vi "Move Stage.vi"() -> ()   [LabVIEW 2016]
uses:
  C:/Program Files/Newport/Piezo Motion Control/Newport AG-UC2-UC8 Applet/Samples/LabVIEW 2009/AgilisCmdLib.dll
  Program Files/Newport/Piezo Motion Control/Newport AG-UC2-UC8 Applet/Samples/LabVIEW 2009/AgilisCmdLib.dll
panel:
  in  "Step speed":i64(ring)=3 items=["Off", "Slow", "Medium", "Fast"]
  in  "Direction":bool
  in  "stop GUI":bool
  in  "Go!":bool
  in  "Stage Address":i32(ring)=3 items=["Dropper"=3, "opposite to dropper"=1, "beside dropper"=2]
  out "error out":errorcluster
  # "In"
  # "Out"
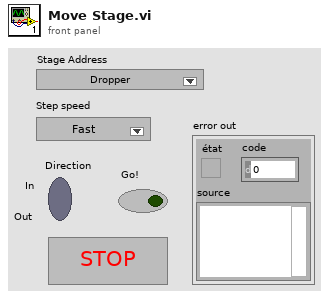
[diagram p1: front panel]
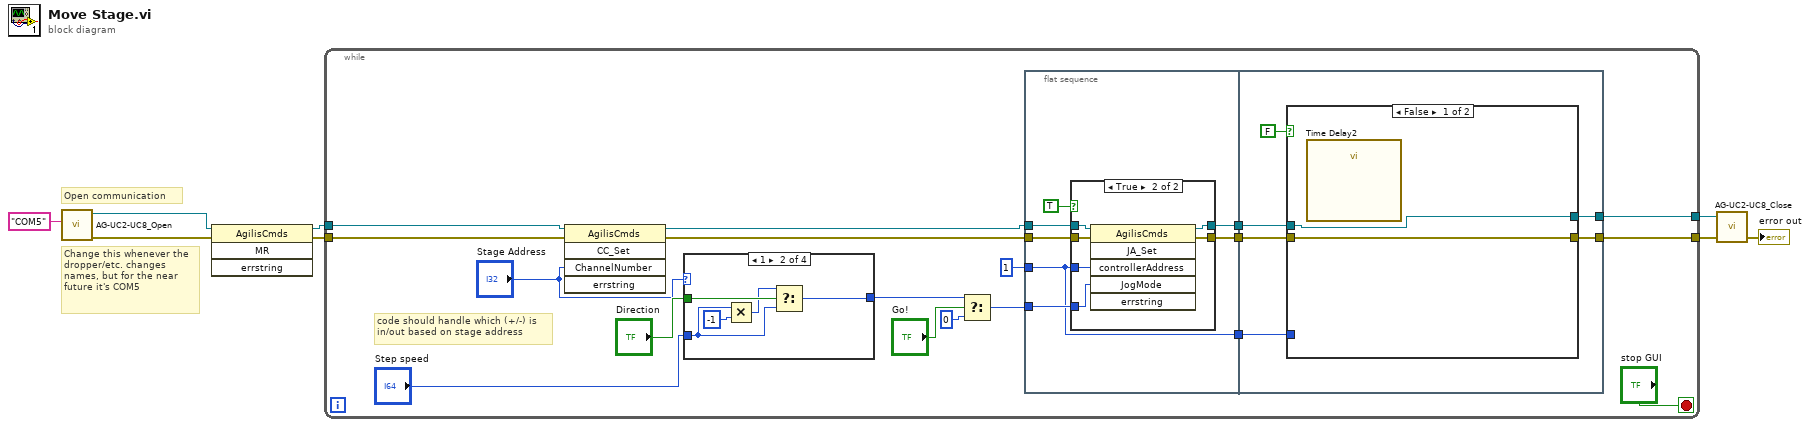
[diagram p0: block diagram]
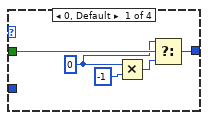
[diagram p2: hidden frame]
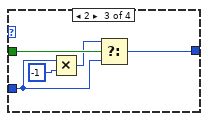
[diagram p3: hidden frame]
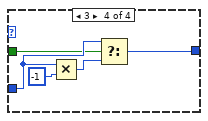
[diagram p4: hidden frame]
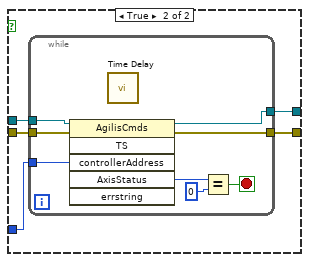
[diagram p6: hidden frame]
diagram:
  # "Change this whenever the dropper/etc. changes names, but for the near future it's COM5"
  # "Open communication"
  n1 = call "AG-UC2-UC8_Open.vi"("Instrument Key IN"="COM5") -> ("error out"=w2:errorcluster, "AG-UC2-UC8 Reference"=w3:refnum<k24>)  [unwired: 3 in, 2 out]
  n2 = invoke class="AgilisCmds" method="MR"(reference=w3, error in=w2) -> (reference out=w4:refnum<k24>, error out=w5:errorcluster)  [unwired: 2 in, 2 out]
  n3 = while {
    tunnel: [w23] -> w7
    tunnel: [w22] -> w6
    tunnel: w4 -> [w17]
    tunnel: w5 -> [w16]
    stop <- "stop GUI" stop-if-true
    # "code should handle which (+/-) is in/out based on stage address"
    n4 = invoke class="AgilisCmds" method="CC_Set"(reference=w17, error in=w16, "ChannelNumber"="Stage Address") -> (reference out=w15:refnum<k24>, error out=w14:errorcluster)  [unwired: 2 in, 3 out]
    n5 = case shown="1" "Stage Address" {
      tunnel: "Step speed" -> [_ w33 w37 w46]
      tunnel: [w29 w35 w39 w43] -> w9
      tunnel: "Direction" -> [w30 w34 w40 w44]
      frame 0, Default {
        w27 = i64 0 ("y")
        n6 = Multiply(x=w27, y=i64 -1) -> (x*y=w28:i32)
        n7 = Select(t=w27, s=w30, f=w28) -> (s? t:f=w29:i64)
      }
      frame 1 {
        n8 = Multiply(x=w33, y=i64 -1) -> (x*y=w32:i32)
        n9 = Select(t=w32, s=w34, f=w33) -> (s? t:f=w35:i64)
      }
      frame 2 {
        n10 = Multiply(x=w37, y=i64 -1) -> (x*y=w38:i32)
        n11 = Select(t=w38, s=w40, f=w37) -> (s? t:f=w39:i64)
      }
      frame 3 {
        n12 = Multiply(x=w46, y=i64 -1) -> (x*y=w42:i32)
        n13 = Select(t=w46, s=w44, f=w42) -> (s? t:f=w43:i64)
      }
    }
    n14 = Select(t=w9, s="Go!", f=i64 0) -> (s? t:f=w18:i64)
    n15 = flat-sequence {
      tunnel: w14 -> [w53]
      tunnel: w15 -> [w52]
      tunnel: 1 ("controllerAddress") -> [w48]
      tunnel: w18 -> [w51]
      tunnel: [w50] -> w26
      tunnel: [w49] -> w25
      tunnel: [w48] -> w21
      tunnel: w26 -> [w67]
      tunnel: w25 -> [w66]
      tunnel: [w65] -> w23
      tunnel: [w64] -> w22
      tunnel: w21 -> [w63]
      frame #0 {
        n16 = case shown="True" TRUE {
          tunnel: w53 -> [w54 w61]
          tunnel: w52 -> [w55 w60]
          tunnel: w48 -> [_ w59]
          tunnel: w51 -> [_ w56]
          tunnel: [w55 w58] -> w50
          tunnel: [w54 w57] -> w49
          frame False {
          }
          frame True {
            n17 = invoke class="AgilisCmds" method="JA_Set"(reference=w60, error in=w61, "controllerAddress"=w59, "JogMode"=w56) -> (reference out=w58:refnum<k24>, error out=w57:errorcluster)  [unwired: 2 in, 4 out]
          }
        }
      }
      frame #1 {
        n18 = case shown="False" FALSE {
          tunnel: w67 -> [w69 w74]
          tunnel: w66 -> [w68 w73]
          tunnel: [w68 w72] -> w65
          tunnel: [w69 w71] -> w64
          tunnel: w63 -> [_ w70]
          frame False {
            n19 = call "Time Delay2"() -> ()  [unwired: 11 in, 1 out]
          }
          frame True {
            n20 = while {
              tunnel: w74 -> [w79]
              tunnel: w73 -> [w78]
              tunnel: [w77] -> w72
              tunnel: [w76] -> w71
              tunnel: w70 -> [w75]
              stop <- w82 stop-if-true
              n21 = invoke class="AgilisCmds" method="TS"(reference=w79, error in=w78, "controllerAddress"=w75) -> (reference out=w76:refnum<k24>, error out=w77:errorcluster, "AxisStatus"=w81:i32)  [unwired: 3 in, 3 out]
              n22 = call "Time Delay"() -> ()  [unwired: 11 in, 1 out]
              n23 = Equal?(x=w81, y=0) -> (x = y?=w82:bool)
            }
          }
        }
      }
    }
  }
  n24 = call "AG-UC2-UC8_Close.vi"("error in (no error)"=w7, "AG-UC2-UC8 Reference"=w6) -> ("Error out"=→"error out":errorcluster)  [unwired: 2 in, 1 out]
